vi "SignalGenerator.vi"() -> ()   [LabVIEW 2017]
uses:
  <vilib>/express/express analysis/Spectral/Block/exnSpectralBlock spectral measurements RMS poly.vi
  <vilib>/express/express analysis/Spectral/Block/exnSpectralBlock spectral measurements RMS DDT.vi
  <vilib>/express/express analysis/Spectral/XNode/ExpressSpectralMeasurementsBlockNode.xnode
panel:
  out "Sine":dynamicdata(graph)
  out "Waveform Graph":dynamicdata(graph)
  in  "Frequency":dbl(knob)=10.1 scale=0.0..22050.0
  in  "On / Off":bool
  in  "stop":bool
  # "Developed by Vincent Claes"
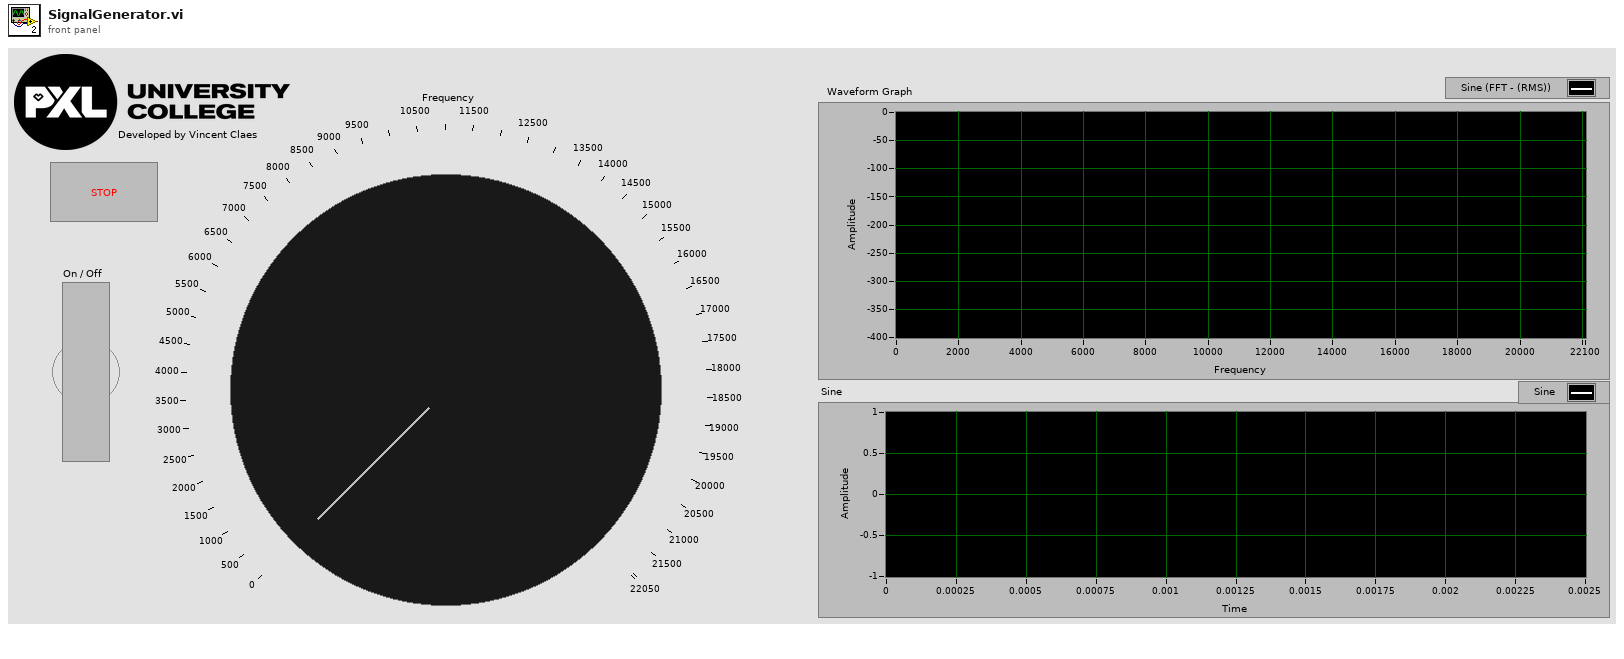
[diagram p1: front panel]
types:
  T1 = cluster{"averaging mode":u16, "weighting mode":u16, "number of averages":u32}
  T2 = cluster{"dB On (F)":bool, "unwrap phase (F)":bool, "convert to degree (F)":bool}
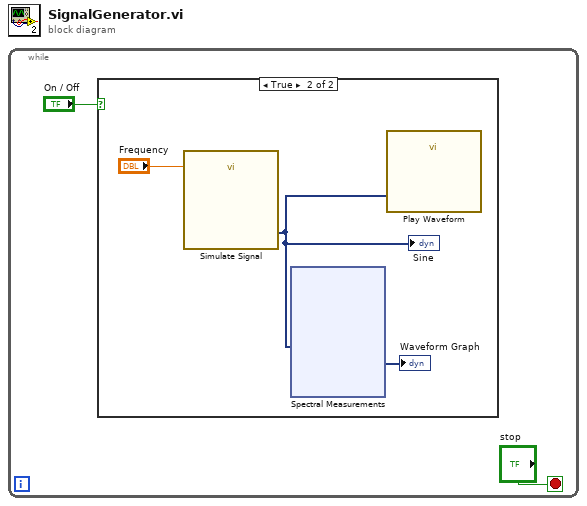
[diagram p0: block diagram]
diagram:
  n1 = while {
    stop <- "stop" stop-if-true
    n2 = case shown="True" "On / Off" {
      frame False {
      }
      frame True {
        n3 = call "Simulate Signal"("Frequency"="Frequency") -> ("Sine"=w4:dynamicdata)  [unwired: 13 in, 1 out]
        "Sine" <- w4
        n4 = xnode "Spectral Measurements"("Signals"=w4) -> ("FFT - (RMS)"=→"Waveform Graph":dynamicdata)  [unwired: 1 in, 2 out]
        n5 = call "Play Waveform"("Data"=w4) -> ()  [unwired: 18 in, 1 out]
      }
    }
  }
